vi "PID Output Rate Limiter.vi"   [LabVIEW 2017]
doc: "This function can be used to specify a maximum rate of change of the controller output. Place this VI immediately after the PID VI in your control application."
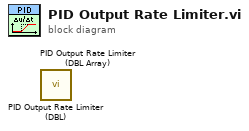
[diagram p0: block diagram]
diagram:
  n1 = call "PID Output Rate Limiter (DBL).vi"() -> ()  [unwired: 8 in, 2 out]
  n2 = call "PID Output Rate Limiter (DBL Array).vi"() -> ()  [unwired: 8 in, 2 out]
